vi "Get Window Size.vi"(0 "VI in":refnum<vi>, 11 "error in (no error)":errorcluster) -> (4 "VI out":refnum<vi>, 8 "Height":i16, 15 "error out":errorcluster)   [LabVIEW 2015]
panel:
  out "Width":i16
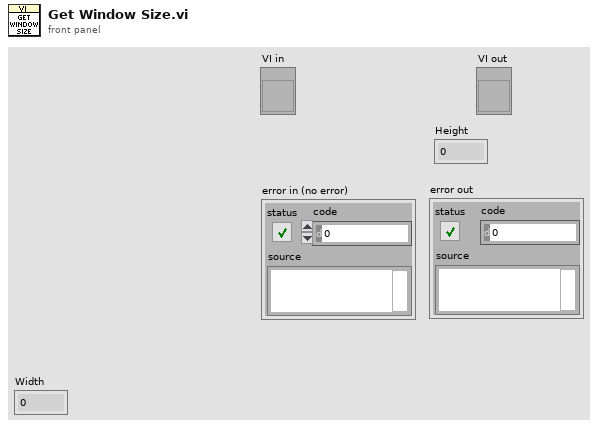
[diagram p1: front panel]
types:
  T1 = typedef "LVRectTypeDef.ctl" = cluster{"Left":i16, "Top":i16, "Right":i16, "Bottom":i16}
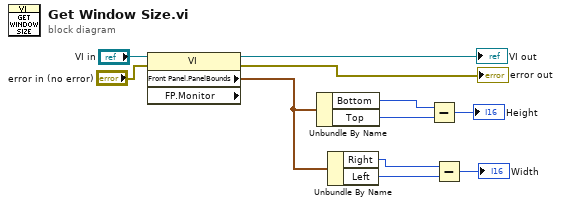
[diagram p0: block diagram]
diagram:
  n1 = property class="VI" props=["Front Panel.PanelBounds", "FP.Monitor"](reference="VI in", error in="error in (no error)") -> (reference out=→"VI out":refnum<vi>, error out=→"error out":errorcluster, "Front Panel.PanelBounds"=w2:T1)  [unwired: 1 out]
  n2 = Unbundle By Name(w2) -> ("Bottom"=w6:i16, "Top"=w8:i16)
  n3 = Unbundle By Name(w2) -> ("Right"=w1:i16, "Left"=w4:i16)
  n4 = Subtract(x=w6, y=w8) -> (x-y=→"Height":i16)
  n5 = Subtract(x=w1, y=w4) -> (x-y=→"Width":i16)
